vi "FTW-Actor-Log-FrameworkEvent.vi"(0 "FTW Actor Instance":refnum<class "FTW-Actor-Instance.lvclass">, 5 "Framework Event":T1, 7 "Event Data":string, 11 "error in":errorcluster) -> (4 "FTW Actor Instance out":refnum<class "FTW-Actor-Instance.lvclass">, 15 "error out":errorcluster)   [LabVIEW 2015, in "FTW-Actor-Instance.lvclass"]
uses:
  FTW-Actor-Instance.lvclass
  FTW-Actor-FrameworkEvent.ctl
  FTW-Actor-Instance.lvclass/FTW-Actor-Instance.ctl
panel:
  # "Inputs"
  # "Outputs"
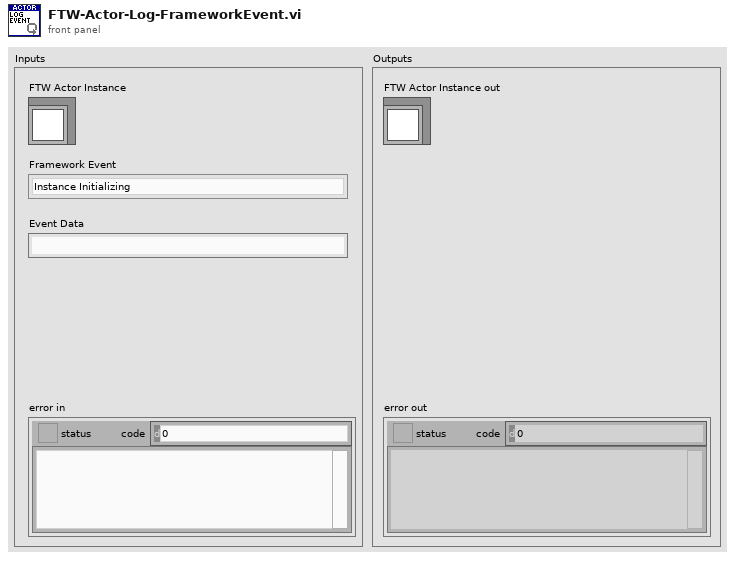
[diagram p1: front panel]
types:
  T1 = typedef "FTW-Actor-Instance.lvclass/FTW-Actor-FrameworkEvent.ctl" = enum16{"Instance Initializing", "Instance Initialized", "Instance Job", "Instance Handle Request", "Instance Shutting Down", "Instance Destroyed"}
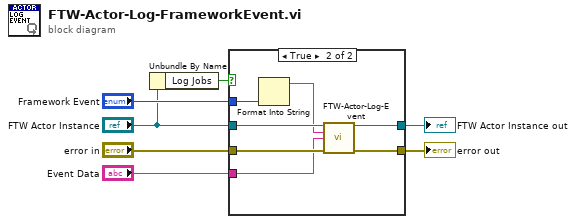
[diagram p0: block diagram]
diagram:
  n1 = Unbundle By Name("FTW Actor Instance") -> ("Log Jobs"=w1:bool)
  n2 = case shown="True" w1 {
    tunnel: "FTW Actor Instance" -> [w9 w16]
    tunnel: [w9 w15] -> w7
    tunnel: "error in" -> [w8 w14]
    tunnel: [w8 w13] -> w6
    tunnel: "Event Data" -> [_ w12]
    tunnel: "Framework Event" -> [_ w11]
    frame False {
    }
    frame True {
      n3 = Format Into String(w11) -> (resulting string=w10:string)  [unwired: 3 in, 1 out]
      n4 = call-dynamic "FTW-Actor-Log-Event.vi"("FTW Actor Instance"=w16, "Event Type"=w10, "Event Data"=w12, "error in"=w14) -> ("FTW Actor Instance out"=w15:refnum<class "FTW-Actor-Instance.lvclass">, "error out"=w13:errorcluster)  [unwired: 10 in]
    }
  }
  "error out" <- w6
  "FTW Actor Instance out" <- w7
